vi "Create Evaluations.vi"(8 "error in (no error)":errorcluster, 11 "IEvaluation in":refnum<class "Skyworks_SpurTest.lvclass">) -> (0 "error out":errorcluster, 2 "Evaluations Out":T1[](array[typedef]) {"Low Limit" format="%#_13g"; "SI Scaling" items=["femto"=-15, "pico"=-12, "nano"=-9, "micro"=-6, "milli"=-3, "percent"=-2, ""=0, "kilo"=3, "mega"=6, "giga"=9, "tera"=12]}, 3 "IEvaluation out":refnum<class "Skyworks_SpurTest.lvclass">)   [LabVIEW 2016, in "SeqAuto Evaluations.lvlib" / "Skyworks_SpurTest.lvclass"]
uses:
  Skyworks_SpurTest.lvclass
  C:/Sequence Automation/Plugins/SeqAuto IEvaluation.lvlibp/SeqAuto IEvaluation.lvclass
  Plugins/TestStand API Tools (TSAT).lvlibp/Evaluation Actions/Includes/Controls/TSAT Evaluation.ctl
  Plugins/TestStand API Tools (TSAT).lvlibp/Evaluation Actions/Includes/Controls/TSAT Eval SI Unit Scaling.ctl
  Plugins/TestStand API Tools (TSAT).lvlibp/Evaluation Actions/Includes/Controls/TSAT Evaluation Type.ctl
  Skyworks_SpurTest.lvclass/Skyworks_SpurTest.ctl
  Plugins/SeqAuto IEvaluation.lvlibp/Read Measurement Name.vi
  Plugins/TestStand API Tools (TSAT).lvlibp/Evaluation Actions/TSAT Evaluation Actions.lvlib
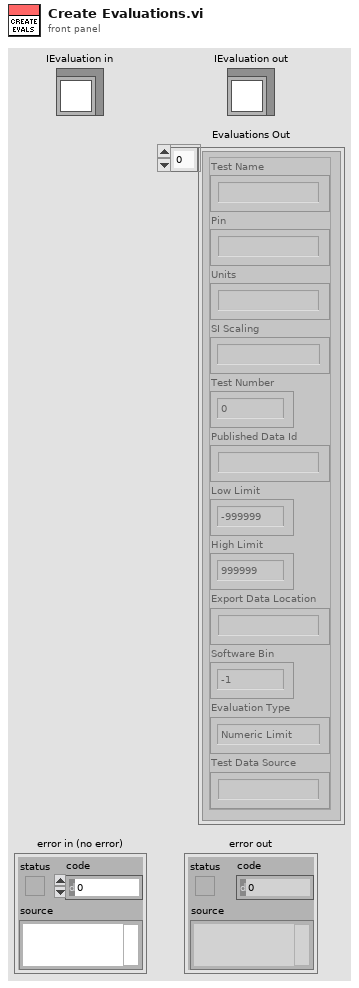
[diagram p1: front panel]
types:
  T1 = typedef "TestStand API Tools (TSAT).lvlibp/TSAT Evaluation Actions.lvlib/TSAT Evaluation.ctl" = cluster{"Test Name":string, "Pin":string, "Units":string, "SI Scaling":T2, "Test Number":i32, "Published Data Id":string, "Low Limit":dbl, "High Limit":dbl, "Export Data Location":string, "Software Bin":i64, "Evaluation Type":T3, "Test Data Source":string}
  T2 = typedef "TestStand API Tools (TSAT).lvlibp/TSAT Evaluation Actions.lvlib/TSAT Eval SI Unit Scaling.ctl" = i16
  T3 = typedef "TestStand API Tools (TSAT).lvlibp/TSAT Evaluation Actions.lvlib/TSAT Evaluation Type.ctl" = enum16{"Numeric Limit", "Pass/Fail", "None"}
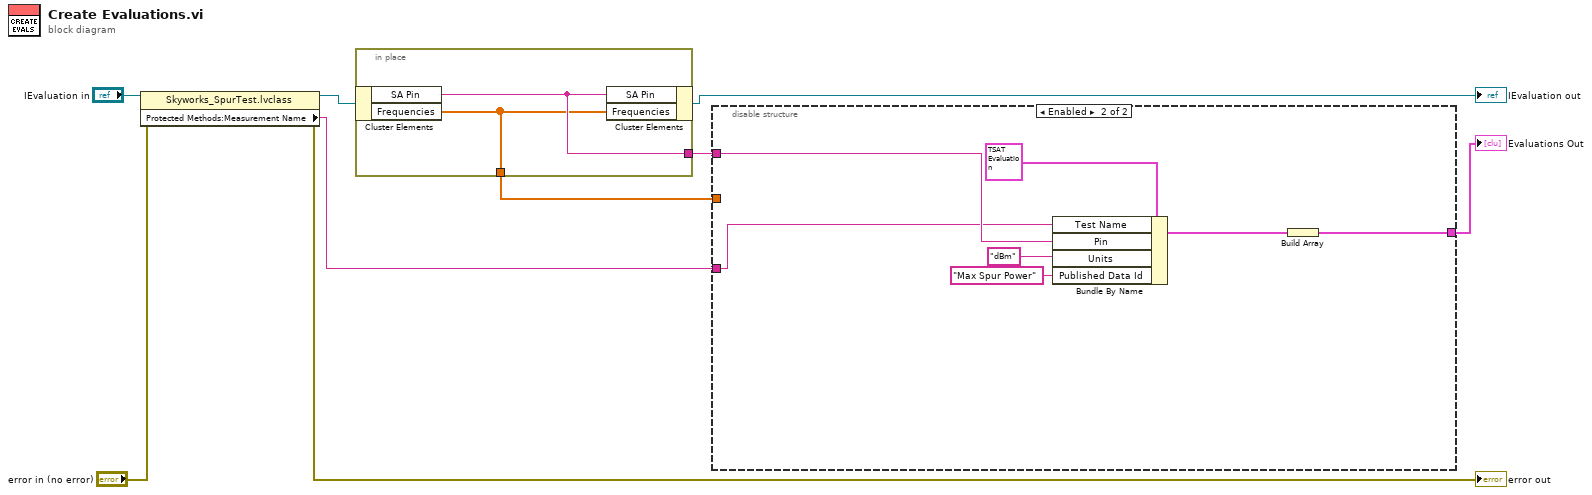
[diagram p0: block diagram]
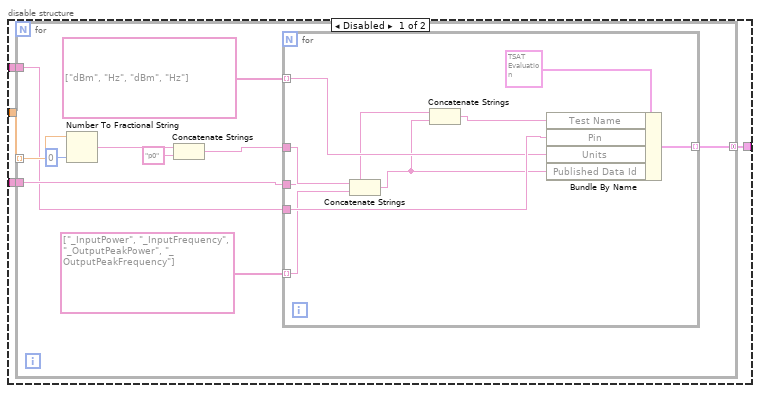
[diagram p2: hidden frame]
diagram:
  n1 = property class="Skyworks_SpurTest.lvclass"(reference="IEvaluation in", error in="error in (no error)") -> (reference out=w6:refnum<class "Skyworks_SpurTest.lvclass">, error out=→"error out":errorcluster, "Protected Methods:Measurement Name"=w2:string)
  n2 = in-place {
    in-place-border: [w11] -> w4
    in-place-border: [w10] -> w3
    n3 = in-place-cluster #1(w6) -> ("SA Pin"=w11:string, "Frequencies"=w10:dbl[])
    n4 = in-place-cluster #1("SA Pin"=w11, "Frequencies"=w10) -> (→"IEvaluation out":refnum<class "Skyworks_SpurTest.lvclass">)
  }
  n5 = disable-structure shown="Enabled" {
    disable-tunnel: w4 -> [w15 w38]
    disable-tunnel: w3 -> [w14 _]
    disable-tunnel: w2 -> [w13 w35]
    disable-tunnel: [w12 w39] -> w1
    frame Disabled {
      n6 = for {
        tunnel: w15 -> [w19]
        tunnel: w14 -> [w24] mode=indexing
        tunnel: w13 -> [w25]
        tunnel: [w16] -> w12 mode=concatenating
        n7 = Number To Fractional String(number=w24, precision (6)=i16 0) -> (F-format string=w23:string)  [unwired: 2 in]
        n8 = Concatenate Strings(w23, "p0" ("string")) -> (w21:string)
        n9 = for {
          tunnel: w25 -> [w29]
          tunnel: w21 -> [w31]
          tunnel: w19 -> [w33]
          tunnel: string[] ["dBm", "Hz", "dBm", "Hz"] -> [w32] mode=indexing
          tunnel: string[] ["_InputPower", "_InputFrequency", "_OutputPeakPower", "_OutputPeakFrequency"] -> [w30] mode=indexing
          tunnel: [w26] -> w16 mode=indexing
          n10 = Concatenate Strings(w31, w30) -> (w28:string)
          n11 = Concatenate Strings(w29, w28) -> (w27:string)
          n12 = Bundle By Name(cluster=T1 {"Test Name"="", "Pin"="", "Units"="", "SI Scaling"=0, "Test Number"=0, "Published Data Id"="", "Low Limit"=-999999.0, "High Limit"=999999.0, "Export Data Location"="", "Software Bin"=-1, "Evaluation Type"=enum."Numeric Limit", "Test Data Source"=""} ("Evaluation"), "Test Name"=w27, "Pin"=w33, "Units"=w32, "Published Data Id"=w28) -> (w26:T1)
        }
      }
    }
    frame Enabled {
      n13 = Bundle By Name(cluster=T1 {"Test Name"="", "Pin"="", "Units"="", "SI Scaling"=0, "Test Number"=0, "Published Data Id"="", "Low Limit"=0.0, "High Limit"=0.0, "Export Data Location"="", "Software Bin"=0, "Evaluation Type"=enum."Numeric Limit", "Test Data Source"=""} ("Evaluation"), "Test Name"=w35, "Pin"=w38, "Units"="dBm", "Published Data Id"="Max Spur Power") -> (w40:T1)
      n14 = Build Array(w40) -> (w39:T1[])
    }
  }
  "Evaluations Out" <- w1
